vi "Update Edge Ports.vi"(0 "Edges In":refnum<class "FSM.Edge.lvclass">[](array[class]), 7 "FSM.Node In":refnum<class "FSM.Node.lvclass">, 11 "Edges":enum16{"Incoming", "Outgoing"}(ring)) -> (4 "Edges Out":refnum<class "FSM.Edge.lvclass">[](array[class]), 8 "FSM.Node thru":refnum<class "FSM.Node.lvclass">)   [LabVIEW 2020, in "FSM.Graph.lvclass"]
uses:
  FSM.Graph.lvclass
  FSM.Edge/FSM.Edge.lvclass
  FSM.Node/FSM.Node.lvclass
  FSM.Node/FSM.Node.lvclass/FSM.Node.ctl
  FSM.Edge/FSM.Edge.lvclass/FSM.Edge.ctl
  FSM.Edge/Read TargetName.vi
  FSM.Edge/Read SourceName.vi
  FSM.Node/Read Name.vi
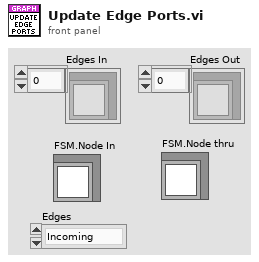
[diagram p1: front panel]
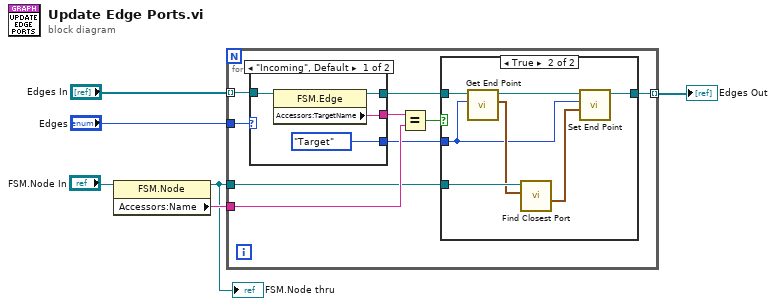
[diagram p0: block diagram]
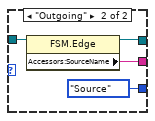
[diagram p3: hidden frame]
diagram:
  n1 = property class="FSM.Node"(reference="FSM.Node In") -> (reference out=w2:refnum<class "FSM.Node.lvclass">, "Accessors:Name"=w3:string)  [unwired: 1 in, 1 out]
  "FSM.Node thru" <- w2
  n2 = for {
    tunnel: "Edges In" -> [w15] mode=indexing
    tunnel: "Edges" -> [w14]
    tunnel: w3 -> [w12]
    tunnel: w2 -> [w8]
    tunnel: [w9] -> w1 mode=indexing
    n3 = case shown="\"Incoming\", Default" w14 {
      tunnel: w15 -> [w27 w31]
      tunnel: [w26 w30] -> w13
      tunnel: [w25 w29] -> w11
      tunnel: [enum16{"Source", "Target"}."Target" ("End") enum16{"Source", "Target"}."Source" ("End")] -> w7
      frame "Incoming", Default {
        n4 = property class="FSM.Edge"(reference=w27) -> (reference out=w25:refnum<class "FSM.Edge.lvclass">, "Accessors:TargetName"=w26:string)  [unwired: 1 in, 1 out]
      }
      frame "Outgoing" {
        n5 = property class="FSM.Edge"(reference=w31) -> (reference out=w29:refnum<class "FSM.Edge.lvclass">, "Accessors:SourceName"=w30:string)  [unwired: 1 in, 1 out]
      }
    }
    n6 = Equal?(x=w13, y=w12) -> (x = y?=w10:bool)
    n7 = case shown="True" w10 {
      tunnel: w11 -> [w16 w22]
      tunnel: [w16 w19] -> w9
      tunnel: w8 -> [_ w23]
      tunnel: w7 -> [_ w17]
      frame False {
      }
      frame True {
        n8 = call "Get End Point.vi"("End"=w17, "FSM.Edge in"=w22) -> ("point"=w21:cluster{"x":i16, "y":i16}, "FSM.Edge out"=w20:refnum<class "FSM.Edge.lvclass">)  [unwired: 7 in, 1 out]
        n9 = call "Find Closest Port.vi"("point"=w21, "FSM.Node in"=w23) -> ("Location"=w18:cluster{"x":i16, "y":i16})  [unwired: 6 in, 3 out]
        n10 = call "Set End Point.vi"("point"=w18, "End"=w17, "FSM.Edge in"=w20) -> ("FSM.Edge out"=w19:refnum<class "FSM.Edge.lvclass">)  [unwired: 7 in, 1 out]
      }
    }
  }
  "Edges Out" <- w1
